vi "ReadRingini.vi"(0 "Data In":T2, 5 "PrintNum":u16 caption="列印數:") -> (2 "PrintName":string, 3 "FMT_out":T6={"formatNo"=1, "x"="25", "y"="10", "Is180Rotation"=FALSE, "IsReflected"=0, "copies"=1}, 4 "Data Out":T2, 6 "GetBIM_out1":T1={"xPosition"="9", "yPosition"="2", "familyName"="Arial", "emSize"=6.0, "printText"="CS-RX110JHA2"}, 8 "GetBIM_out2":T1={"xPosition"="9", "yPosition"="2", "familyName"="Arial", "emSize"=6.0, "printText"="CS-RX110JHA2"}, 10 "GetBIM_out3":T1={"xPosition"="9", "yPosition"="2", "familyName"="Arial", "emSize"=6.0, "printText"="CS-RX110JHA2"}, 13 "QRC_out":T5={"startX"="2", "startY"="3", "cellSize"=3, "inoutMode"=1, "maskNumber"=9, "errorLevel"=1, "terminator"=2, "modelNumber"=2, "strData"="設定機種品番"} {"terminator" items=["NUL"=1, "ETX"=2, "EOT"=3]}, 14 "PRT_out":T4={"quantity"=1, "cutUnit"=0, "fixedNO"=1}, 15 "GetBIM_out4":T1={"xPosition"="9", "yPosition"="2", "familyName"="Arial", "emSize"=6.0, "printText"="CS-RX110JHA2"})   [LabVIEW 2014]
uses:
  controls/FMT.ctl
  controls/GetBIM.ctl
  controls/QRC.ctl
  controls/PRT.ctl
  controls/Data1.ctl
  controls/Payjson.ctl
  <vilib>/Utility/file.llb/Read From Spreadsheet File (string).vi
panel:
  in  "Prnum":string
  out "COMPNTID":string
  in  "BarCode":string
  in  "Date":string
  in  "HinBan":string
  in  "ModelName":string
  in  "PRT":T4={"quantity"=1, "cutUnit"=0, "fixedNO"=1}
  in  "QRC":T5={"startX"="2", "startY"="3", "cellSize"=3, "inoutMode"=1, "maskNumber"=9, "errorLevel"=1, "terminator"=2, "modelNumber"=2, "strData"="設定機種品番"} {"terminator" items=["NUL"=1, "ETX"=2, "EOT"=3]}
  in  "GetBIM":T1={"xPosition"="9", "yPosition"="2", "familyName"="Arial", "emSize"=6.0, "printText"="CS-RX110JHA2"}
  in  "FMT":T6={"formatNo"=1, "x"="25", "y"="10", "Is180Rotation"=FALSE, "IsReflected"=0, "copies"=1}
  out "GetBIM_1":string[](array[string])
  out "FMT":string[](array[string])
  out "all rows":string[][](array[string])
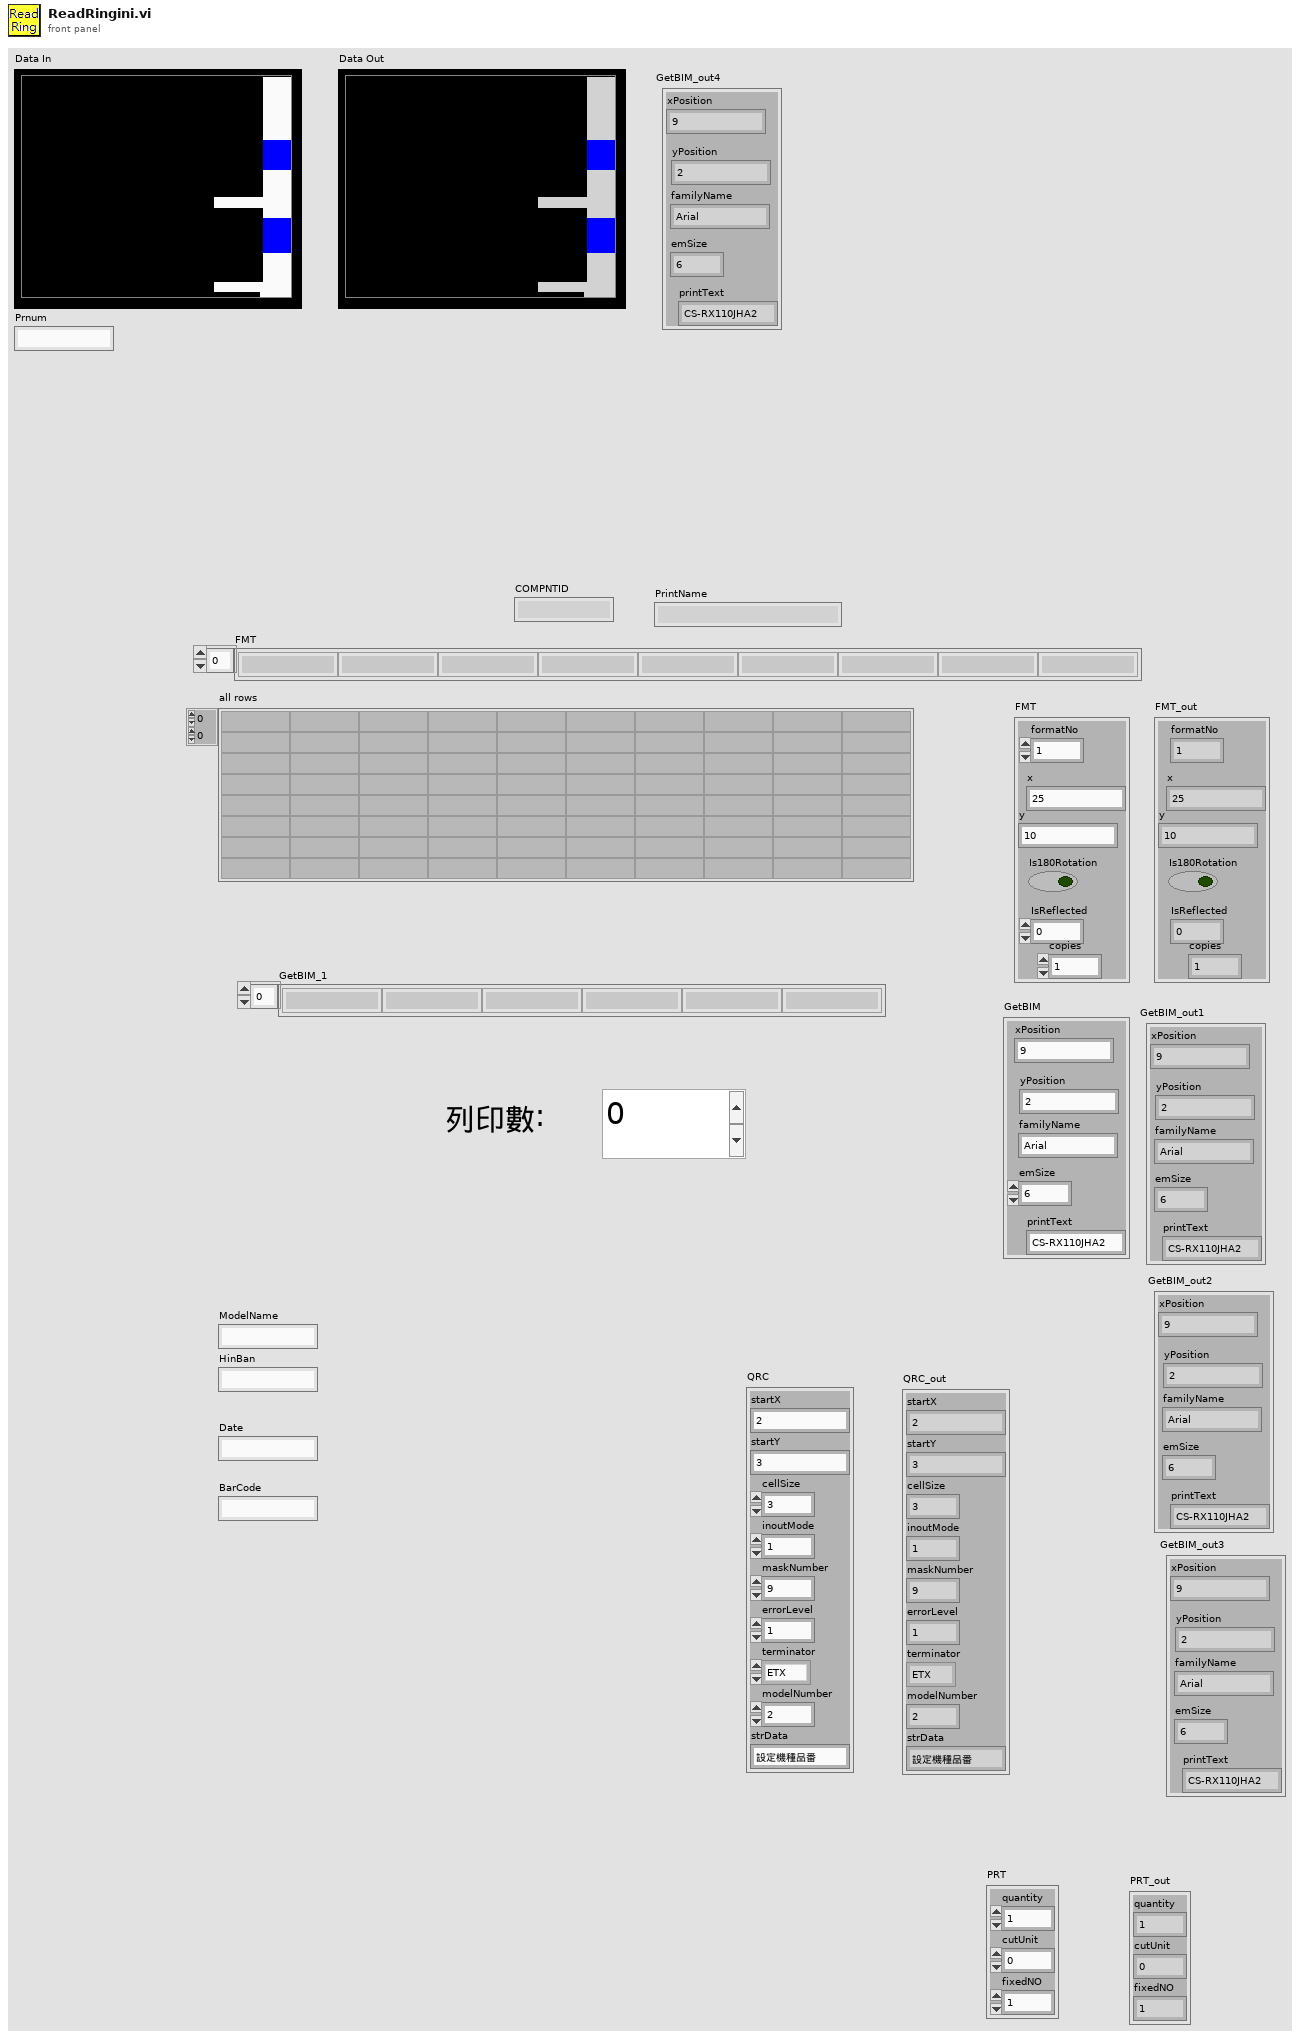
[diagram p1: front panel]
types:
  T1 = typedef "GetBIM.ctl" = cluster{"xPosition":string, "yPosition":string, "familyName":string, "emSize":sgl, "printText":string}
  T2 = typedef "Data1.ctl" = cluster{"Date":string, "BarCode1":string, "BarCode2":string, "BarCode3":string, "Message":string, "OK Count":u16, "NG Count":u16, "Total Count":u16, "ModelData":string[][], "OK&NG":bool, "COM1":refnum<visa-resource-name>, "COM2":refnum<visa-resource-name>, "IO":i32, "Time":u32, "TCP":refnum<k5>, "TCP 2":refnum<k5>, "COM1 2":refnum<visa-resource-name>, "CheckNum":string, "BarCode1_1":string, "BarCode2_1":string, "BarCode3_1":string, "日期":string, "機種":string, "機號":string, "商品條碼1":string, "OK_1":string, "OK":string, "NG":string, "NG_1":string, "Total":string, "Total_1":string, "ClaerTime":u32, "Pjson":T3, "LotNo":string[], "CheckParsArray":string[], "BarCode4":string, "BarCode4_1":string, "商品條碼2":string, "BarCode5":string, "BarCode5_1":string, "商品條碼3":string, "ReScanNG":i32, "NGTimeCT":u32}
  T3 = typedef "Payjson.ctl" = cluster{"DEPT":string, "LINE":string, "STANO":string, "WORKNO":string, "PRODSN":string, "COMPNTID":string, "COMPNTLOT":string, "COMPNTSN":string, "USEDQTY":i16, "OPDATE":string, "OPUSER":string, "RECVDATE":string, "MMODU":string}[]
  T4 = typedef "PRT.ctl" = cluster{"quantity":i32, "cutUnit":i32, "fixedNO":i32}
  T5 = typedef "QRC.ctl" = cluster{"startX":string, "startY":string, "cellSize":i32, "inoutMode":i32, "maskNumber":i32, "errorLevel":i32, "terminator":i32, "modelNumber":i32, "strData":string}
  T6 = typedef "FMT.ctl" = cluster{"formatNo":i32, "x":string, "y":string, "Is180Rotation":bool, "IsReflected":u8, "copies":u8}
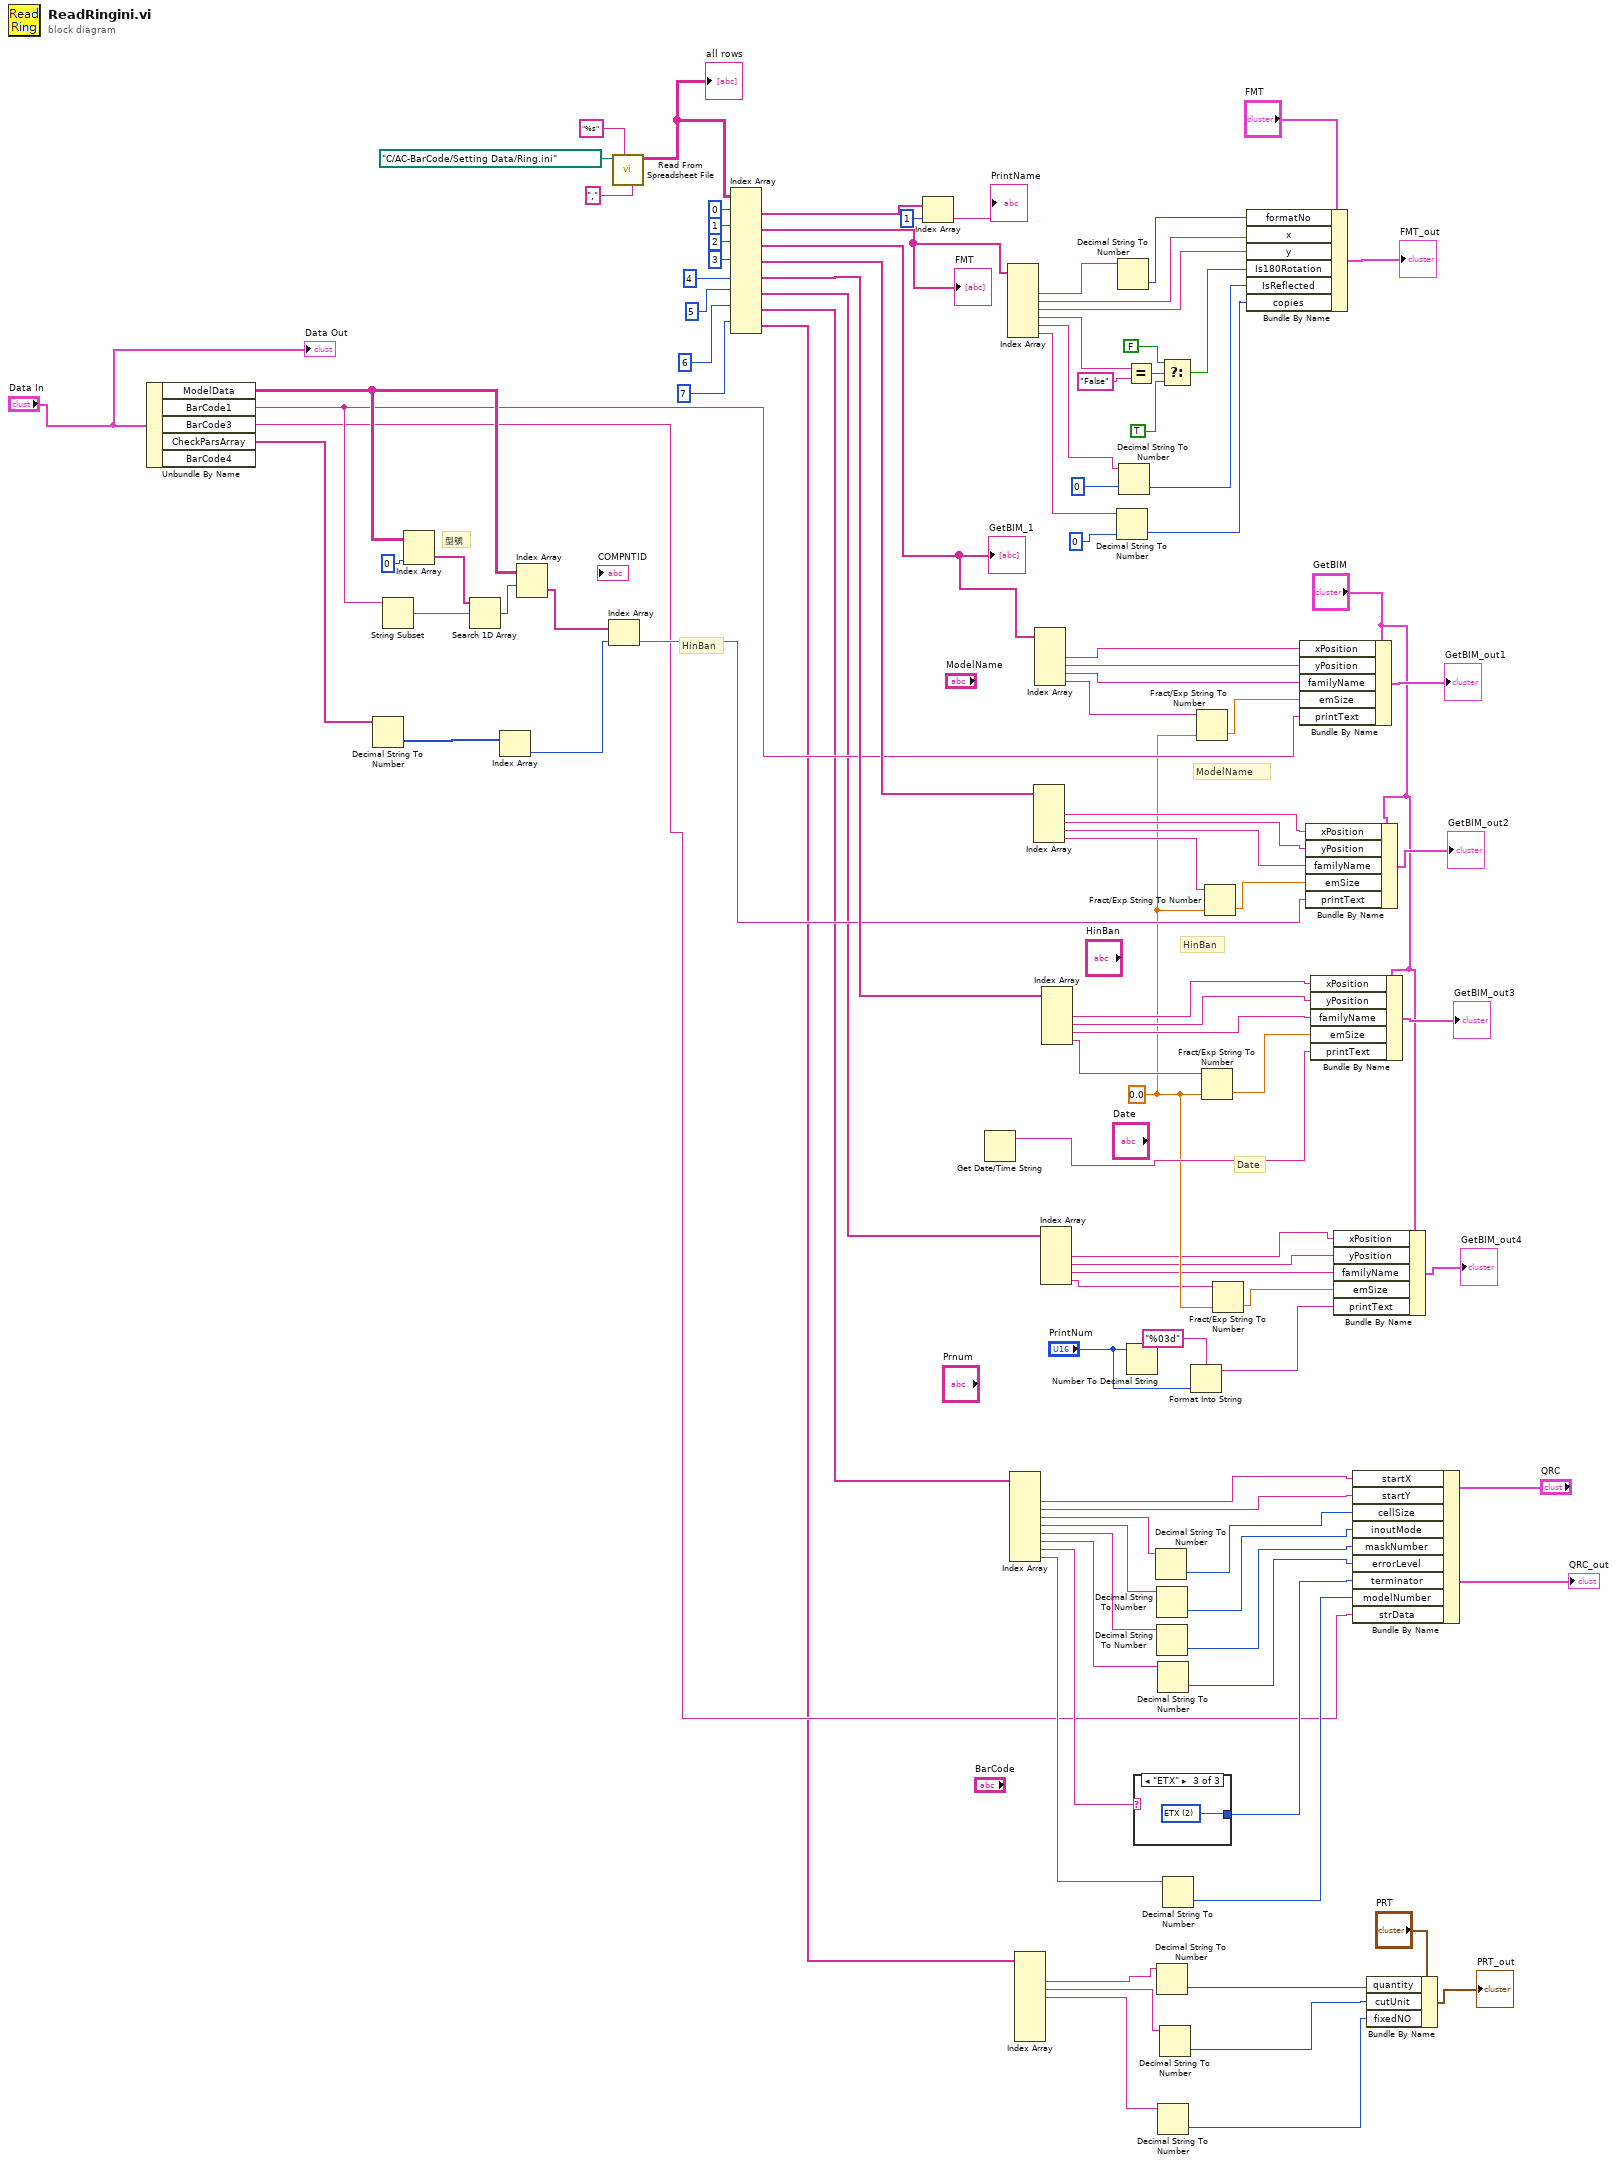
[diagram p0: block diagram]
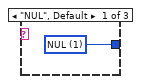
[diagram p2: hidden frame]
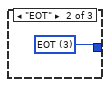
[diagram p3: hidden frame]
diagram:
  w11 = sgl 0.0 ("emSize")
  # "HinBan"
  # "Date"
  # "HinBan"
  # "ModelName"
  # "型號"
  n1 = Unbundle By Name("Data In") -> ("ModelData"=w25:string[][], "BarCode1"=w21:string, "BarCode3"=w18:string, "CheckParsArray"=w17:string[])  [unwired: 1 out]
  n2 = Decimal String To Number(string=w17) -> (number=w23:i32[])  [unwired: 2 in, 1 out]
  n3 = String Subset(string=w21) -> (substring=w27:string)  [unwired: 2 in]
  n4 = Index Array(array=w25, index (col)=0 ("disabled index (col)")) -> (element=w28:string[])  [unwired: 1 in]
  n5 = Search 1D Array(1D array=w28, element=w27) -> (index of element=w26:i32)  [unwired: 1 in]
  n6 = Index Array(array=w23) -> (element=w22:i32)  [unwired: 1 in]
  n7 = Index Array(array=w25, index (row)=w26) -> (element=w24:string[])  [unwired: 1 in]
  n8 = Index Array(array=w24, index=w22) -> (element=w20:string)
  n9 = call-poly <vilib>:"Read From Spreadsheet File.vi"("delimiter (\\t)"="," ("delimiter (\\t)"), "format (%s)"="%s", "file path (dialog if empty)"=path "C:/AC-BarCode/Setting Data/Ring.ini") -> ("all rows"=w104:string[][])  [unwired: 4 in, 4 out]
  "all rows" <- w104
  n10 = Index Array(array=w104, index (row) #1=0 ("index (row)"), index (row) #2=1 ("index (row)"), index (row) #3=2 ("index (row)"), index (row) #4=3 ("index (row)"), index (row) #5=4 ("index (row)"), index (row) #6=5 ("disabled index (col)"), index (row) #7=6 ("index (row)"), index (row) #8=7 ("index (row)")) -> (element #1=w102:string[], element #2=w96:string[], element #3=w77:string[], element #4=w63:string[], element #5=w56:string[], element #6=w12:string[], element #7=w14:string[], element #8=w15:string[])  [unwired: 8 in]
  "FMT" <- w96
  "GetBIM_1" <- w77
  n11 = Index Array(array=w102, index=1) -> (element=→"PrintName":string)
  n12 = Get Date/Time String() -> (date string=w19:string)  [unwired: 3 in, 1 out]
  n13 = Index Array(array=w96) -> (element #2=w94:string, element #3=w92:string, element #4=w91:string, element #5=w89:string, element #6=w84:string, element #7=w83:string)  [unwired: 7 in, 1 out]
  n14 = Index Array(array=w14) -> (element #2=w52:string, element #3=w51:string, element #4=w50:string, element #5=w48:string, element #6=w46:string, element #7=w44:string, element #8=w42:string, element #9=w40:string)  [unwired: 9 in, 1 out]
  n15 = Index Array(array=w15) -> (element #2=w35:string, element #3=w34:string, element #4=w30:string)  [unwired: 9 in, 6 out]
  n16 = Index Array(array=w63) -> (element #2=w70:string, element #3=w69:string, element #4=w68:string, element #5=w67:string)  [unwired: 5 in, 1 out]
  n17 = Index Array(array=w77) -> (element #2=w76:string, element #3=w75:string, element #4=w74:string, element #5=w73:string)  [unwired: 5 in, 1 out]
  n18 = Index Array(array=w12) -> (element #2=w7:string, element #3=w6:string, element #4=w5:string, element #5=w4:string)  [unwired: 5 in, 1 out]
  n19 = Index Array(array=w56) -> (element #2=w62:string, element #3=w61:string, element #4=w60:string, element #5=w59:string)  [unwired: 5 in, 1 out]
  n20 = Decimal String To Number(string=w83, default (0L)=u8 0) -> (number=w79:u8)  [unwired: 1 in, 1 out]
  n21 = Decimal String To Number(string=w94) -> (number=w93:i32)  [unwired: 2 in, 1 out]
  n22 = Decimal String To Number(string=w84, default (0L)=u8 0) -> (number=w81:u8)  [unwired: 1 in, 1 out]
  n23 = Equal?(x=w89, y="False") -> (x = y?=w90:bool)
  n24 = Number To Decimal String(number="PrintNum") -> ()  [unwired: 1 in, 1 out]
  n25 = case shown="\"ETX\"" w42 {
    tunnel: [w108 w109 w110] -> w41
    frame "NUL", Default {
      w108 = 1 items=["NUL"=1, "ETX"=2, "EOT"=3] ("terminator")
    }
    frame "EOT" {
      w109 = 3 items=["NUL"=1, "ETX"=2, "EOT"=3] ("terminator")
    }
    frame "ETX" {
      w110 = 2 items=["NUL"=1, "ETX"=2, "EOT"=3] ("terminator")
    }
  }
  n26 = Decimal String To Number(string=w50) -> (number=w49:i32)  [unwired: 2 in, 1 out]
  n27 = Decimal String To Number(string=w48) -> (number=w47:i32)  [unwired: 2 in, 1 out]
  n28 = Decimal String To Number(string=w46) -> (number=w45:i32)  [unwired: 2 in, 1 out]
  n29 = Decimal String To Number(string=w35) -> (number=w33:i32)  [unwired: 2 in, 1 out]
  n30 = Decimal String To Number(string=w44) -> (number=w43:i32)  [unwired: 2 in, 1 out]
  n31 = Decimal String To Number(string=w30) -> (number=w31:i32)  [unwired: 2 in, 1 out]
  n32 = Decimal String To Number(string=w34) -> (number=w32:i32)  [unwired: 2 in, 1 out]
  n33 = Select(t=FALSE, s=w90, f=TRUE) -> (s? t:f=w85:bool)
  n34 = Decimal String To Number(string=w40) -> (number=w39:i32)  [unwired: 2 in, 1 out]
  n35 = Format Into String(format string="%03d", "PrintNum") -> (resulting string=w1:string)  [unwired: 2 in, 1 out]
  n36 = Fract/Exp String To Number(string=w73, default (0 dbl)=w11) -> (number=w72:sgl)  [unwired: 2 in, 1 out]
  n37 = Fract/Exp String To Number(string=w59, default (0 dbl)=w11) -> (number=w58:sgl)  [unwired: 2 in, 1 out]
  n38 = Fract/Exp String To Number(string=w67, default (0 dbl)=w11) -> (number=w66:sgl)  [unwired: 2 in, 1 out]
  n39 = Fract/Exp String To Number(string=w4, default (0 dbl)=w11) -> (number=w10:sgl)  [unwired: 2 in, 1 out]
  n40 = Bundle By Name(cluster="FMT", "formatNo"=w93, "x"=w92, "y"=w91, "Is180Rotation"=w85, "IsReflected"=w81, "copies"=w79) -> (→"FMT_out":T6)
  n41 = Bundle By Name(cluster="GetBIM", "xPosition"=w76, "yPosition"=w75, "familyName"=w74, "emSize"=w72, "printText"=w21) -> (→"GetBIM_out1":T1)
  n42 = Bundle By Name(cluster="GetBIM", "xPosition"=w70, "yPosition"=w69, "familyName"=w68, "emSize"=w66, "printText"=w20) -> (→"GetBIM_out2":T1)
  n43 = Bundle By Name(cluster="GetBIM", "xPosition"=w62, "yPosition"=w61, "familyName"=w60, "emSize"=w58, "printText"=w19) -> (→"GetBIM_out3":T1)
  n44 = Bundle By Name(cluster="GetBIM", "xPosition"=w7, "yPosition"=w6, "familyName"=w5, "emSize"=w10, "printText"=w1) -> (→"GetBIM_out4":T1)
  n45 = Bundle By Name(cluster="QRC", "startX"=w52, "startY"=w51, "cellSize"=w49, "inoutMode"=w47, "maskNumber"=w45, "errorLevel"=w43, "terminator"=w41, "modelNumber"=w39, "strData"=w18) -> (→"QRC_out":T5)
  n46 = Bundle By Name(cluster="PRT", "quantity"=w33, "cutUnit"=w32, "fixedNO"=w31) -> (→"PRT_out":T4)
  "Data Out" <- "Data In"
